vi "Setup.vi"(5 "Protocol selection\n(appended)":T1 {"Mode" items=["Modbus-1", "3"]}, 7 "protocol selection ref":refnum<vi>, 8 "error in (no error)":errorcluster, 9 "search":bool, 10 "Comm master cluster in":T4={"Main event var"=refnum, "VIRef"=refnum, "Data path"=path "", "Reads"=0, "total number of UUT"=0, "FF refnum"={"Handle1"=0, "Handle2"=0}, "FF device id list"=[], "MODBUS resource name"="", "MODBUS Serial Parameters"={"Mode"=enum."RTU", "Default Slave Address"=0, "MODBUS timeout"=0, "Baud Rate"=0, "Parity"=0, "Flow Control"=0}, "Profibus resource name"="", "Profibus Communication ref.:"=0, "HART resource name"="", "HART long addresses (array)"=[], "Comm relay session"="", "Comm UI event"=refnum, "Write Interval (s)"=5.0, "DMM_QUEUE"=refnum, "POWER_QUEUE"=refnum, "\nTHERM_QUEUE"=refnum, "\nCOMM_QUEUE"=refnum, "TIMING_QUEUE"=refnum, "MAIN_QUEUE"=refnum, "Log path"=path ""} {"Write Interval (s)" min=0.1 max=1000.0 step=0.1}, 11 "HART in":refnum<class "HART.lvclass">) -> (0 "error out":errorcluster, 3 "HART out":refnum<class "HART.lvclass">)   [LabVIEW 2016, in "HART.lvclass"]
uses:
  HART.lvclass
  MASTER_OPC.ctl
  Typedef/event var.ctl
  Typedef/Comm ui action type.ctl
  Typedef/Comm_State_enum.ctl
  Typedef/state var.ctl
  Typedef/Array_of_Comm_mode_and_address_types.ctl
  Typedef/Comm_mode_and_address_type.ctl
  Typedef/Comm_mode_type_combo.ctl
  Typedef/Protocol_enum_type.ctl
  HART.lvclass/HART.ctl
  Protocol Class/Protocol.lvclass
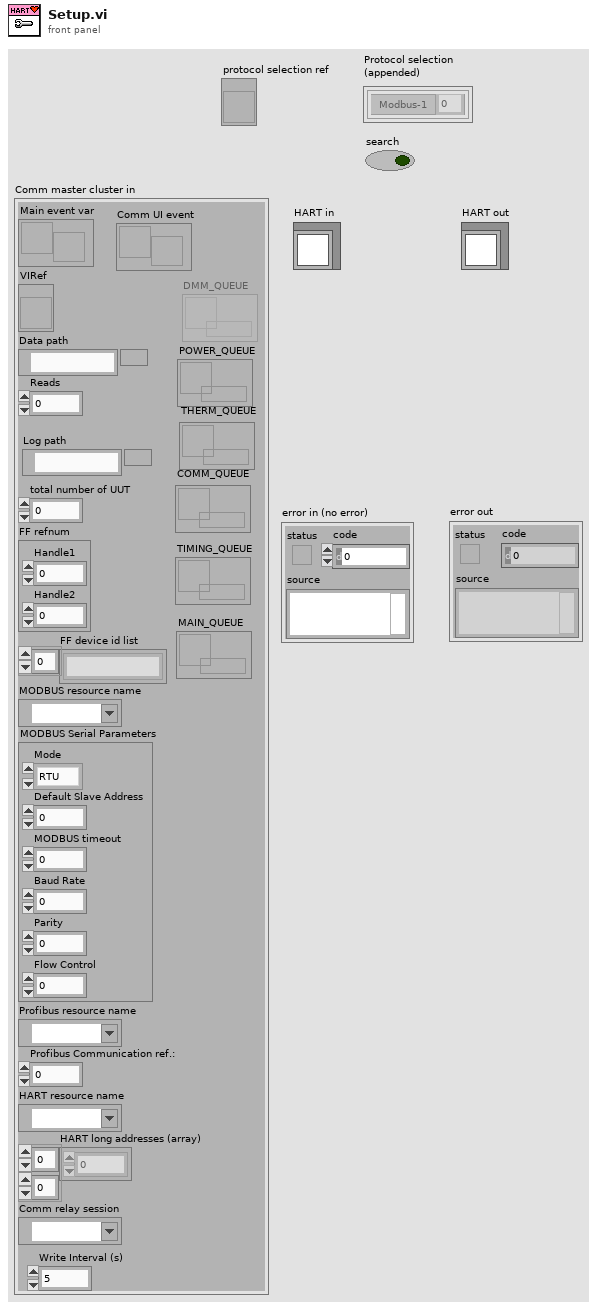
[diagram p1: front panel]
types:
  T1 = typedef "Array_of_Comm_mode_and_address_types.ctl" = T2[]
  T2 = typedef "Comm_mode_and_address_type.ctl" = cluster{"address":i32, "Mode":T3}
  T3 = typedef "Comm_mode_type_combo.ctl" = u16
  T4 = typedef "MASTER_OPC.ctl" = cluster{"Main event var":refnum<user-event>, "VIRef":refnum<vi>, "Data path":path, "Reads":i32, "total number of UUT":i32, "FF refnum":cluster{"Handle1":u32, "Handle2":u32}, "FF device id list":string[], "MODBUS resource name":refnum<visa-resource-name>, "MODBUS Serial Parameters":cluster{"Mode":enum16{"RTU", "ASCII"}, "Default Slave Address":u8, "MODBUS timeout":u32, "Baud Rate":u32, "Parity":u16, "Flow Control":u16}, "Profibus resource name":refnum<visa-resource-name>, "Profibus Communication ref.:":u8, "HART resource name":refnum<visa-resource-name>, "HART long addresses (array)":u8[][], "Comm relay session":refnum<k15>, "Comm UI event":refnum<user-event>, "Write Interval (s)":dbl, "DMM_QUEUE":refnum<queue>, "POWER_QUEUE":refnum<queue>, "\nTHERM_QUEUE":refnum<queue>, "\nCOMM_QUEUE":refnum<queue>, "TIMING_QUEUE":refnum<queue>, "MAIN_QUEUE":refnum<queue>, "Log path":path}
  T5 = typedef "Protocol_enum_type.ctl" = enum16{"None", "MODBUS", "HART", "Fieldbus", "Profibus DP", "Profibus PA", "DeviceNET", "USB"}
  T6 = enum16{"Connect whole bus", "Connect individual UUTs", "Connect none"}
  T7 = cluster{"Long address":u8[], "Short address":i32, "Switch index":i32}
  T8 = cluster{"Long address":u8[], "Short address":i32, "Switch index":i32}[]
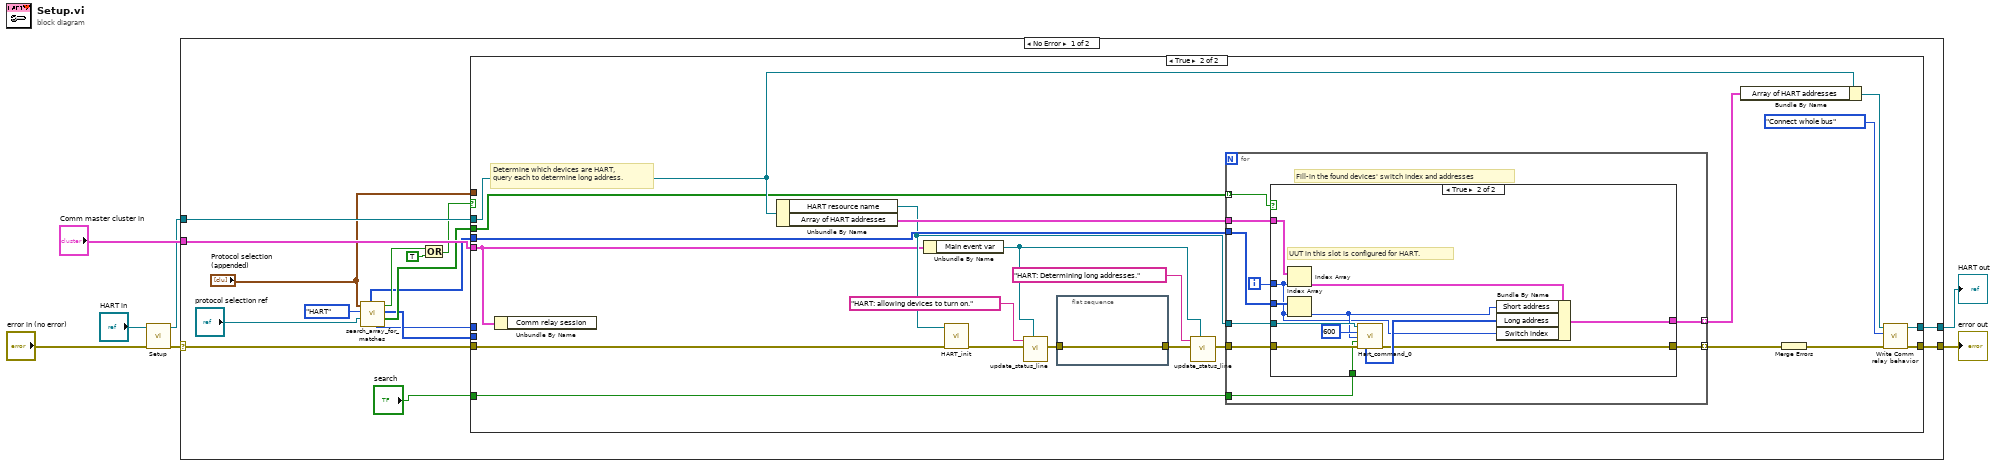
[diagram p0: block diagram]
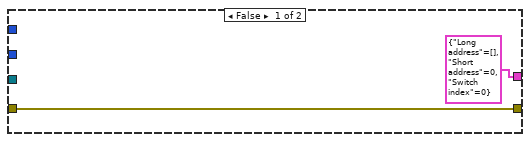
[diagram p3: hidden frame]
diagram:
  n1 = call-parent "Setup.vi"("error in (no error)"="error in (no error)", "Protocol in"="HART in") -> ("error out"=w5:errorcluster, "Protocol out"=w1:refnum<class "HART.lvclass">)  [unwired: 8 in]
  n2 = case shown="No Error" w5 {
    selector: w5 -> [w16 w72]
    tunnel: [w17 w72] -> w4
    tunnel: w1 -> [w20 w73]
    tunnel: [w18 w73] -> w3
    tunnel: "Comm master cluster in" -> [w19 _]
    frame No Error {
      n3 = call "search_array_for_matches.vi"("protocol selection ref"="protocol selection ref", "Protocol enum"=Protocol_enum_type."HART", "appended array"="Protocol selection\n(appended)") -> ("Array of exists"=w14:bool[], "array of indexes"=w12:i32[], "exists?"=w23:bool, "Switch Row"=w11:i32, "all addresses"=w13:i32[])  [unwired: 3 in, 1 out]
      n4 = Or(x=w23, y=TRUE) -> (x .or. y?=w10:bool)
      n5 = case shown="True" w10 {
        tunnel: w13 -> [_ w47]
        tunnel: w20 -> [w25 w45]
        tunnel: [w25 w31] -> w18
        tunnel: w19 -> [_ w33]
        tunnel: [w24 w29] -> w17
        tunnel: w16 -> [w24 w26]
        tunnel: "Protocol selection\n(appended)" -> [_ _]
        tunnel: w14 -> [_ w34]
        tunnel: w12 -> [_ _]
        tunnel: w11 -> [_ _]
        tunnel: "search" -> [_ w27]
        frame False {
          # "No HART devices present in the enabled devices."
        }
        frame True {
          # "Determine which devices are HART, \nquery each to determine long address."
          n6 = Unbundle By Name(w33) -> ()  [unwired: 1 out]
          n7 = Unbundle By Name(w45) -> ("HART resource name"=w37:refnum<visa-resource-name>, "Array of HART addresses"=w46:T8)
          n8 = Unbundle By Name(w33) -> ("Main event var"=w42:refnum<user-event>)
          n9 = call "HART_init.vi"("error in"=w26, "resource name"=w37) -> ("error out"=w39:errorcluster)  [unwired: 9 in]
          n10 = call "update_status_line.vi"("user event"=w42, "error in (no error)"=w39, "message"="HART: allowing devices to turn on.") -> ("error out"=w40:errorcluster)  [unwired: 7 in, 1 out]
          n11 = flat-sequence {
            tunnel: w40 -> [w48]
            tunnel: [w48] -> w43
            frame #0 {
            }
          }
          n12 = call "update_status_line.vi"("user event"=w42, "error in (no error)"=w43, "message"="HART: Determining long addresses.") -> ("error out"=w36:errorcluster)  [unwired: 7 in, 1 out]
          n13 = for {
            tunnel: w47 -> [w55]
            tunnel: w37 -> [w57]
            tunnel: w46 -> [w56]
            tunnel: [w54] -> w44 mode=indexing
            tunnel: w36 -> [w53]
            tunnel: [w52] -> w35 mode=indexing
            tunnel: w34 -> [w51] mode=indexing
            tunnel: w27 -> [w49]
            i -> [w50]
            # "Fill-in the found devices' switch index and addresses"
            n14 = case shown="True" w51 {
              tunnel: w57 -> [_ w70]
              tunnel: w56 -> [_ w69]
              tunnel: w55 -> [_ w67]
              tunnel: [T7 {"Long address"=[], "Short address"=0, "Switch index"=0} ("Hart address") w66] -> w54
              tunnel: w53 -> [w58 w65]
              tunnel: [w58 w64] -> w52
              tunnel: w50 -> [_ w61]
              tunnel: w49 -> [_ w60]
              frame False {
              }
              frame True {
                # "UUT in this slot is configured for HART."
                n15 = Index Array(array=w69, index=w61) -> (element=w63:T7)
                n16 = Index Array(array=w67, index=w61) -> (element=w62:i32)
                n17 = call "Hart_command_0.vi"("VISA resource name"=w70, "milliseconds to wait"=u32 600, "Short address"=w62, "search"=w60, "error in (no error)"=w65) -> ("Address (array)"=w68:u8[], "error out"=w64:errorcluster)  [unwired: 4 in, 5 out]
                n18 = Bundle By Name(cluster=w63, "Short address"=w62, "Long address"=w68, "Switch index"=w61) -> (w66:T7)
              }
            }
          }
          n19 = Bundle By Name(cluster=w45, "Array of HART addresses"=w44) -> (w32:refnum<class "HART.lvclass">)
          n20 = Merge Errors(w35) -> (w30:errorcluster)
          n21 = call-dynamic "Write Comm relay behavior.vi"("error in (no error)"=w30, "Comm relay behavior"=T6."Connect whole bus", "Protocol in"=w32) -> ("error out"=w29:errorcluster, "Protocol out"=w31:refnum<class "HART.lvclass">)  [unwired: 7 in]
        }
      }
    }
    frame Error {
    }
  }
  "error out" <- w4
  "HART out" <- w3
